vi "Demo.vi"() -> ()   [LabVIEW 2020, in "Untitled Library 1.lvlib"]
uses:
  Untitled Library 1.lvlib
panel:
  out "error out":errorcluster
  in  "输入数据(十进制)":string="123456789"
  in  "波特率":u32=19200
  in  "串口号":refnum<visa-resource-name>="COM7"
  out "发送的数据":string
  out "错误输出 4":errorcluster caption="错误输出"
  out "错误输出 3":errorcluster caption="错误输出"
  out "错误输出 2":errorcluster caption="错误输出"
  in  "发送":bool
  in  "停止":bool
  out "反馈":string[](array[string])
  out "错误输出":errorcluster
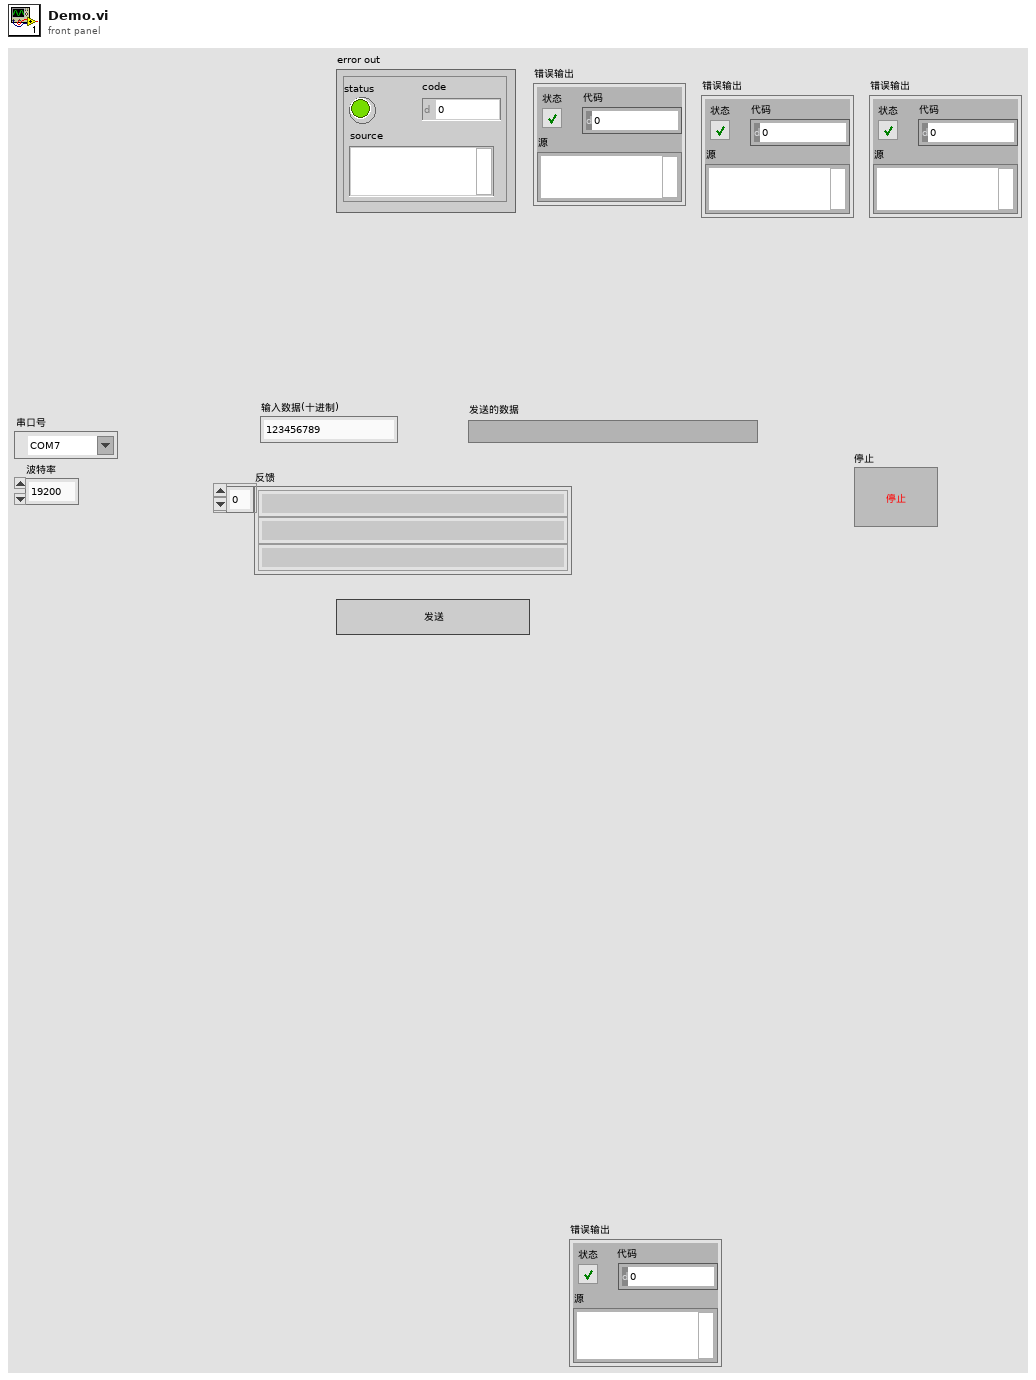
[diagram p1: front panel]
types:
  T1 = enum16{"Open", "Close", "ClearBuffer", "Send", "Read", "SendWaitRead"}
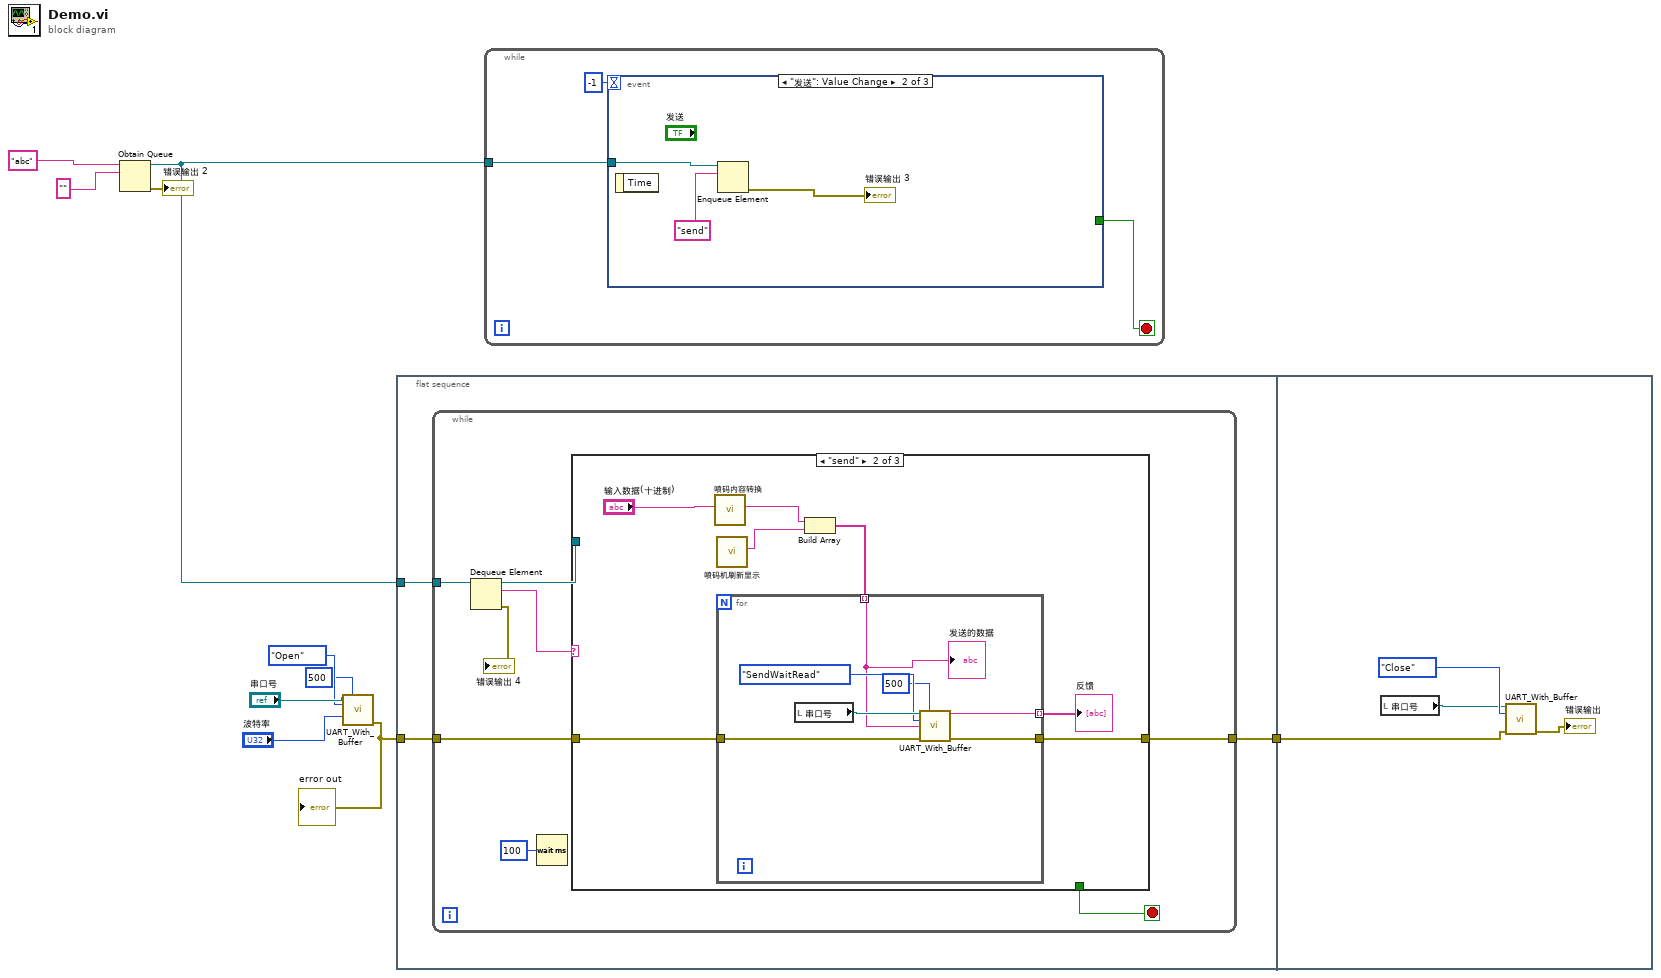
[diagram p0: block diagram]
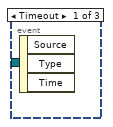
[diagram p2: hidden frame]
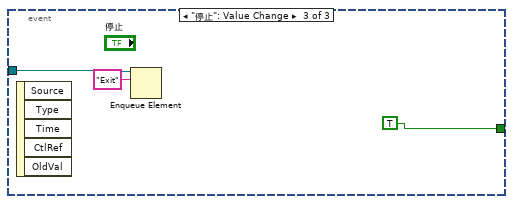
[diagram p3: hidden frame]
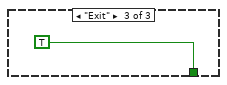
[diagram p5: hidden frame]
diagram:
  n1 = Obtain Queue(name (unnamed)="abc" ("名称（未命名）"), element data type="" ("名称（未命名）")) -> (queue out=w10:refnum<queue>, error out=→"错误输出 2":errorcluster)  [unwired: 3 in, 1 out]
  n2 = call "UART_With_Buffer.vi"("COM"="串口号", "Timeout (ms)"=u32 500, "Function"=T1."Open", "Baudrate"="波特率") -> ("error out"=w3:errorcluster)  [unwired: 10 in, 1 out]
  "error out" <- w3
  n3 = flat-sequence {
    tunnel: w10 -> [w13]
    tunnel: w3 -> [w12]
    tunnel: [w11] -> w2
    tunnel: w2 -> [w37]
    frame #0 {
      n4 = while {
        tunnel: w13 -> [w21]
        tunnel: w12 -> [w15]
        tunnel: [w14] -> w11
        stop <- w19 stop-if-true
        n5 = Dequeue Element(queue=w21) -> (queue out=w20:refnum<queue>, element=w17:string, error out=→"错误输出 4":errorcluster)  [unwired: 2 in, 1 out]
        n6 = Wait (ms)(milliseconds to wait=u32 100 ("等待时间（毫秒）")) -> ()  [unwired: 1 out]
        n7 = case shown="\"send\"" w17 {
          tunnel: w20 -> [_ _ _]
          tunnel: [_ _ TRUE] -> w19
          tunnel: w15 -> [_ w28 _]
          tunnel: [_ w26 _] -> w14
          frame "假", Default {
          }
          frame "send" {
            n8 = call "喷码内容转换.vi"("输入数据(十进制)"="输入数据(十进制)") -> ("输出数据(十六进制)"=w23:string)  [unwired: 10 in]
            n9 = call "喷码机刷新显示.vi"() -> ("刷新显示(16H)"=w22:string)  [unwired: 11 in]
            n10 = Build Array(w23, w22) -> (w24:string[])
            n11 = for {
              tunnel: w24 -> [w30] mode=indexing
              tunnel: w28 -> [w34]
              tunnel: [w32] -> w27 mode=indexing
              tunnel: [w31] -> w26
              n12 = local read "串口号"() -> (w35:refnum<visa-resource-name>)
              n13 = call "UART_With_Buffer.vi"("COM"=w35, "Timeout (ms)"=u32 500, "Function"=T1."SendWaitRead", "Send"=w30, "error in (no error)"=w34) -> ("ReceiveString"=w32:string, "error out"=w31:errorcluster)  [unwired: 9 in]
              "发送的数据" <- w30
            }
            "反馈" <- w27
          }
          frame "Exit" {
          }
        }
      }
    }
    frame #1 {
      n14 = local read "串口号"() -> (w39:refnum<visa-resource-name>)
      n15 = call "UART_With_Buffer.vi"("COM"=w39, "Function"=T1."Close", "error in (no error)"=w37) -> ("error out"=→"错误输出":errorcluster)  [unwired: 11 in, 1 out]
    }
  }
  n16 = while {
    tunnel: w10 -> [w43]
    stop <- w42 stop-if-true
    n17 = event shown="[1] \"发送\": Value Change" {
      selector: _ -> [_ _ _]
      dyn-events: _ -> [_ _ _]
      timeout: -1 -> [_ _ _]
      tunnel: w43 -> [_ w46 w49]
      tunnel: [_ _ TRUE] -> w42
      event Timeout {
        n18 = event-data() -> ()  [unwired: 1 in, 3 out]
      }
      event "发送": Value Change {
        n19 = event-data() -> ()  [unwired: 1 in, 1 out]
        n20 = Enqueue Element(queue=w46, element="send" ("元素")) -> (error out=→"错误输出 3":errorcluster)  [unwired: 2 in, 2 out]
      }
      event "停止": Value Change {
        n21 = event-data() -> ()  [unwired: 1 in, 5 out]
        n22 = Enqueue Element(queue=w49, element="Exit" ("元素")) -> ()  [unwired: 2 in, 3 out]
      }
    }
  }
